vi "Dispose.vi"(8 "error in (no error)":errorcluster, 11 "Redis TCP Client in":refnum<class "Redis TCP Client.lvclass">) -> (0 "error out":errorcluster)   [LabVIEW 2019, in "Redis Client for LabVIEW.lvlib" / "Redis TCP Client.lvclass"]
uses:
  Redis TCP Client.lvclass
  Redis TCP Client.lvclass/Redis TCP Client.ctl
  lib/RESP3-for-LabVIEW/RESP3/RESP3 Parser/RESP3 Parser.lvclass
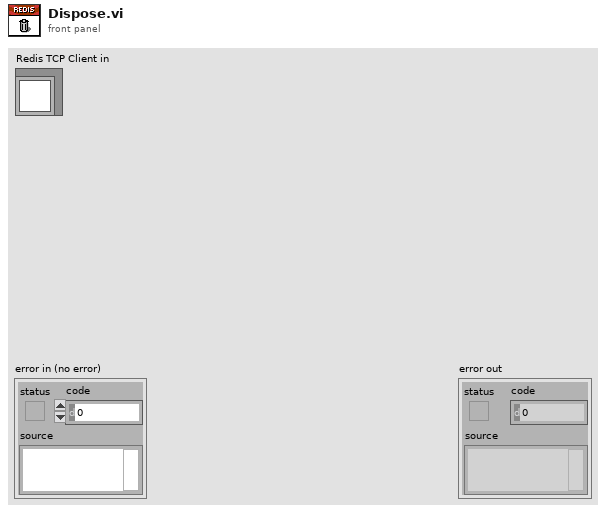
[diagram p1: front panel]
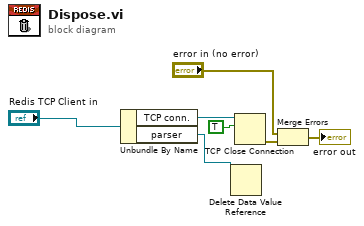
[diagram p0: block diagram]
diagram:
  n1 = Unbundle By Name("Redis TCP Client in") -> ("TCP conn."=w6:refnum<k5>, "parser"=w1:refnum<data-value>)
  n2 = Delete Data Value Reference(data value reference=w1) -> ()  [unwired: 1 in, 2 out]
  n3 = TCP Close Connection(connection ID=w6, abort (F)=TRUE) -> (error out=w5:errorcluster)  [unwired: 1 in, 1 out]
  n4 = Merge Errors("error in (no error)", w5) -> (→"error out":errorcluster)
